vi "TCP Data Stream.vi"(0 "Address":string="localhost", 1 "Port":u16=2055 min=1025 step=1, 2 "Data IN":dbl[][](array[numeric]), 3 "String IN":string, 5 "Error IN":errorcluster, 6 "Mode":T1, 9 "Write String (F)":bool) -> (14 "Data OUT":dbl[][](array[numeric]), 15 "New Data?":bool, 16 "Connected?":bool, 17 "String OUT":string, 19 "Error OUT":errorcluster)   [LabVIEW 2019]
uses:
  Real-Time/Controls/TCP Data Stream Mode.ctl
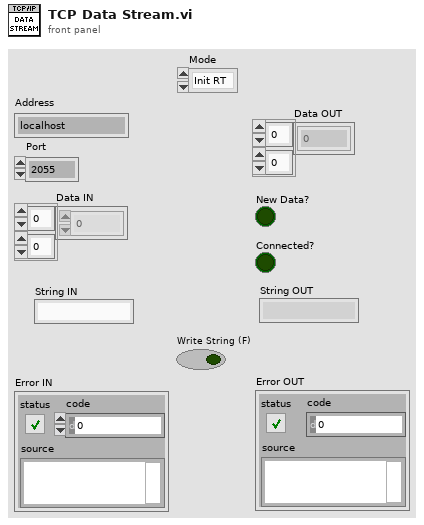
[diagram p1: front panel]
types:
  T1 = typedef "TCP Data Stream Mode.ctl" = enum16{"Init RT", "Init PC", "Connect RT", "Connect PC", "Write Data", "Read Data", "Close"}
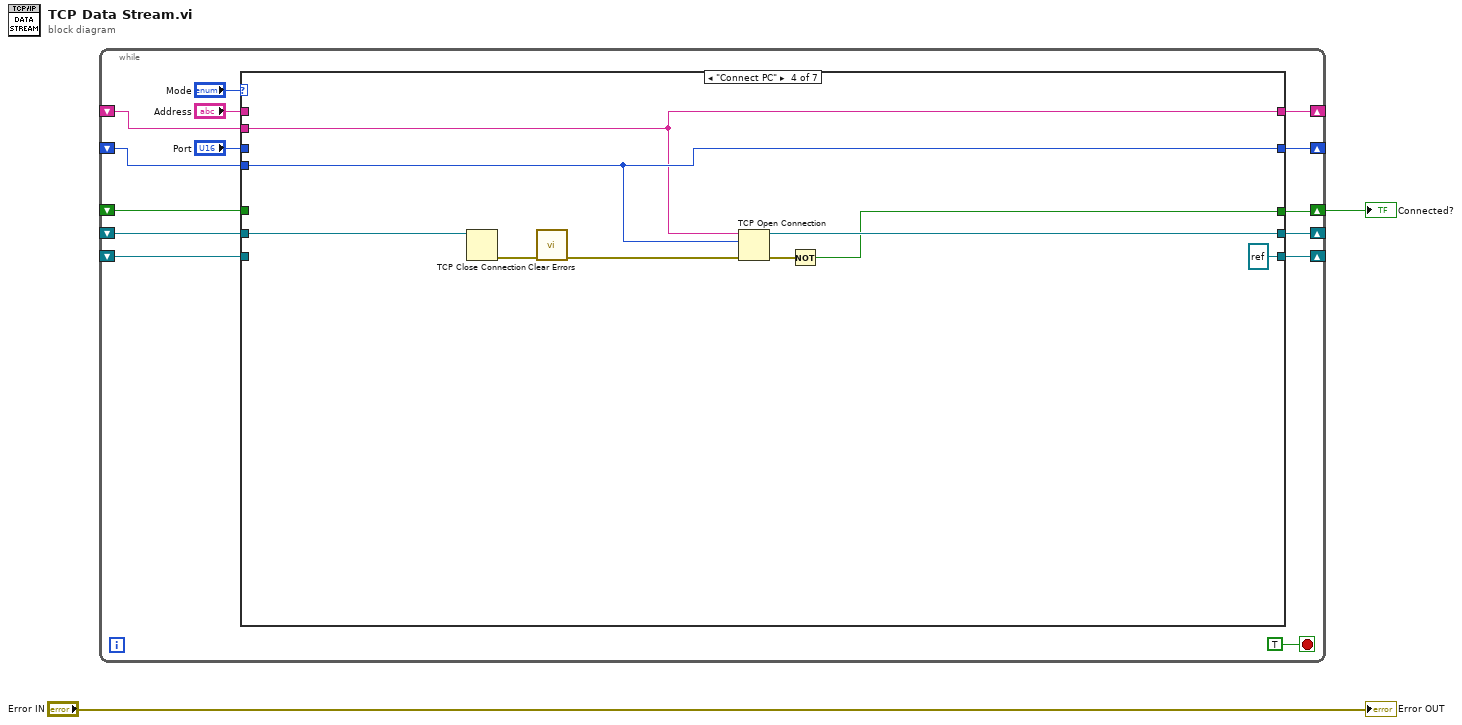
[diagram p0: block diagram]
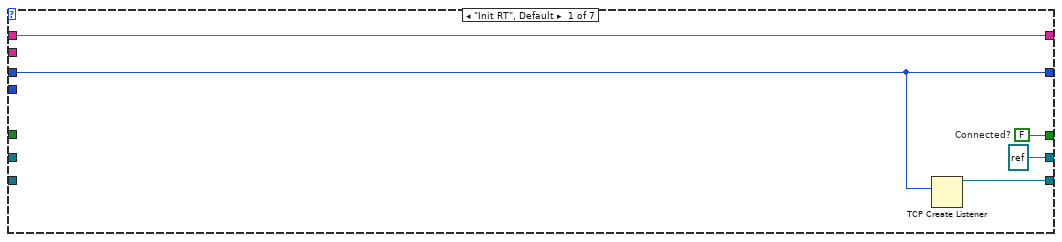
[diagram p2: hidden frame]
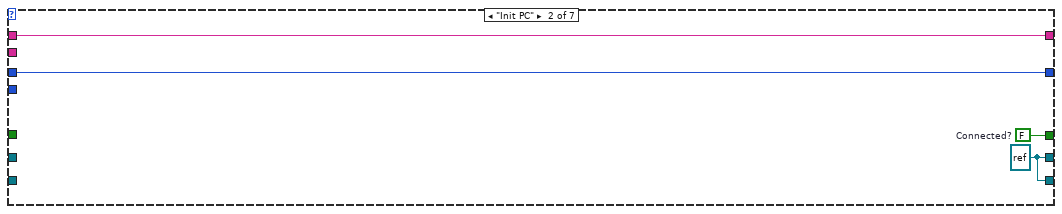
[diagram p3: hidden frame]
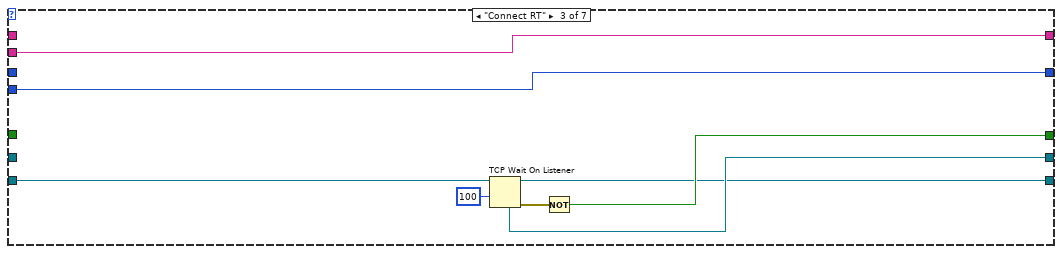
[diagram p4: hidden frame]
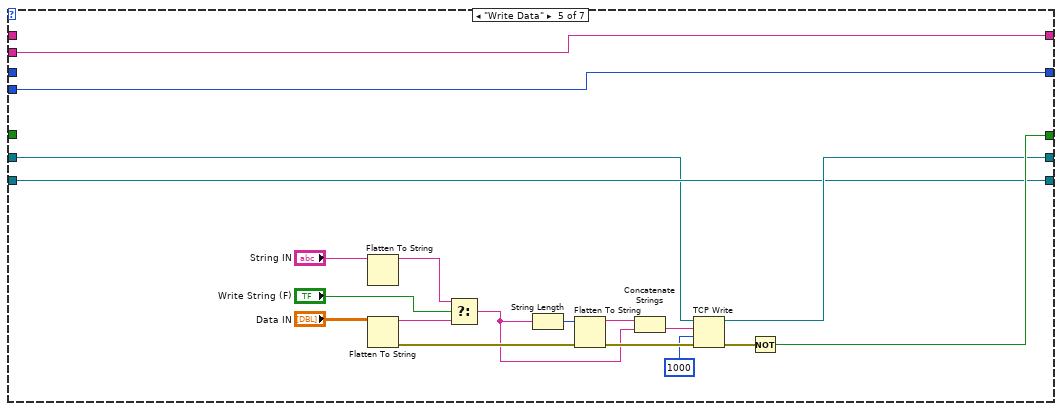
[diagram p5: hidden frame]
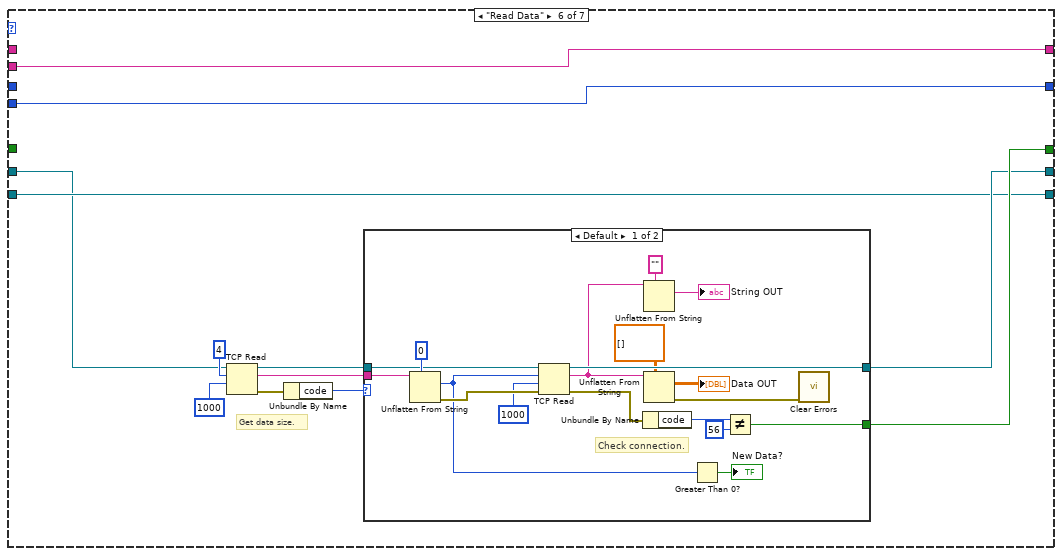
[diagram p6: hidden frame]
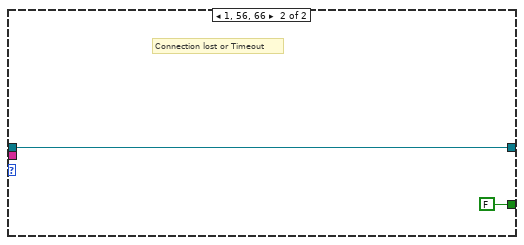
[diagram p7: hidden frame]
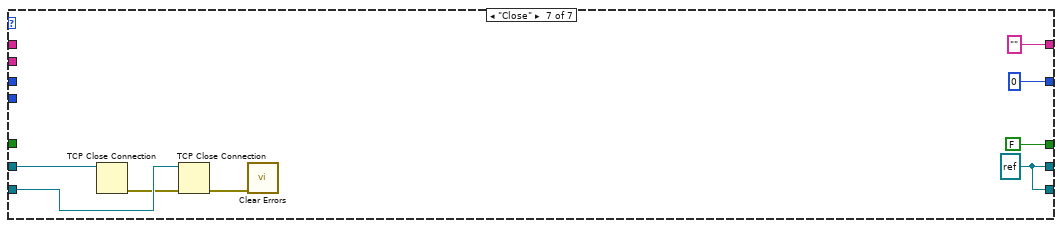
[diagram p8: hidden frame]
diagram:
  n1 = while {
    shift-right: [w13] -> _
    shift-left: _ -> [w8]
    shift-right: [w11] -> _
    shift-left: _ -> [w7]
    shift-right: [w10] -> w2
    shift-left: _ -> [w9]
    shift-right: [w6] -> _
    shift-left: _ -> [w5]
    shift-right: [w4] -> _
    shift-left: _ -> [w3]
    stop <- TRUE stop-if-true
    n2 = case shown="\"Connect PC\"" "Mode" {
      tunnel: [w21 w25 w27 w37 w60 w72 "" ("Address")] -> w13
      tunnel: "Address" -> [w21 w25 _ _ _ _ _]
      tunnel: [w19 w24 w28 w38 w61 w73 u16 0 ("Port")] -> w11
      tunnel: "Port" -> [w19 w24 _ _ _ _ _]
      tunnel: [w20 w23 w31 w40 w59 w71 FALSE ("Client")] -> w10
      tunnel: w9 -> [_ _ _ _ _ _ _]
      tunnel: w8 -> [_ _ w27 w37 w60 w72 _]
      tunnel: w7 -> [_ _ w28 w38 w61 w73 _]
      tunnel: [refnum<k5> refnum ("connection ID") w22 w30 w41 w58 w70 w98] -> w6
      tunnel: w5 -> [_ _ _ w36 w45 w62 w97]
      tunnel: [w17 w22 w29 refnum<k5> refnum ("connection ID") w57 w69 w98] -> w4
      tunnel: w3 -> [_ _ w32 _ w57 w69 w96]
      frame "Init RT", Default {
        w20 = FALSE  # Connected?
        n3 = TCP Create Listener(10:w19) -> (3:w17:refnum<k5>)  [unwired: 4 in, 2 out]
      }
      frame "Init PC" {
        w22 = refnum<k5> refnum ("connection ID")
        w23 = FALSE  # Connected?
      }
      frame "Connect RT" {
        n4 = TCP Wait On Listener(9:100 ("timeout ms (wait forever: -1)"), 11:w32) -> (0:w33:errorcluster, 3:w29:refnum<k5>, 4:w30:refnum<k5>)  [unwired: 2 in, 2 out]
        n5 = Not(x=w33) -> (.not. x?=w31:bool)
      }
      frame "Connect PC" {
        n6 = TCP Close Connection(connection ID=w36) -> (error out=w35:errorcluster)  [unwired: 2 in, 1 out]
        n7 = call <vilib>:"Clear Errors.vi"("error in (no error)"=w35) -> ("error out"=w34:errorcluster)  [unwired: 5 in, 1 out]
        n8 = TCP Open Connection(address=w37, remote port or service name=w38, error in (no error)=w34) -> (connection ID=w41:refnum<k5>, error out=w42:errorcluster)  [unwired: 2 in]
        n9 = Not(x=w42) -> (.not. x?=w40:bool)
      }
      frame "Write Data" {
        n10 = Flatten To String(anything="String IN") -> (data string=w47:string)  [unwired: 1 in, 4 out]
        n11 = Flatten To String(anything="Data IN") -> (data string=w48:string, error out=w55:errorcluster)  [unwired: 1 in, 3 out]
        n12 = Select(t=w47, s="Write String (F)", f=w48) -> (s? t:f=w46:string)
        n13 = String Length(string=w46) -> (length=w53:i32)
        n14 = Flatten To String(anything=w53, error in (no error)=w55) -> (data string=w54:string, error out=w52:errorcluster)  [unwired: 3 out]
        n15 = Concatenate Strings(w54, w46) -> (w51:string)
        n16 = TCP Write(connection ID=w45, data in=w51, error in (no error)=w52, 9:1000 ("timeout ms (25000)")) -> (connection ID out=w58:refnum<k5>, error out=w56:errorcluster)  [unwired: 1 out]
        n17 = Not(x=w56) -> (.not. x?=w59:bool)
      }
      frame "Read Data" {
        # "Get data size."
        n18 = TCP Read(connection ID=w62, bytes to read=4, 9:1000 ("timeout ms (25000)")) -> (connection ID out=w67:refnum<k5>, data out=w66:string, error out=w65:errorcluster)  [unwired: 1 in, 1 out]
        n19 = Unbundle By Name(w65) -> ("code"=w64:i32)
        n20 = case shown="Default" w64 {
          tunnel: [w78 FALSE] -> w71
          tunnel: [w84 w93] -> w70
          tunnel: w67 -> [w89 w93]
          tunnel: w66 -> [w88 _]
          frame Default {
            # "Check connection."
            n21 = Unflatten From String(type=0 ("bytes to read"), binary string=w88) -> (value=w81:i32, error out=w91:errorcluster)  [unwired: 2 in, 2 out]
            n22 = TCP Read(connection ID=w89, bytes to read=w81, error in (no error)=w91, 9:1000 ("timeout ms (25000)")) -> (connection ID out=w84:refnum<k5>, data out=w76:string, error out=w85:errorcluster)  [unwired: 1 out]
            n23 = Unbundle By Name(w85) -> ("code"=w87:i32)
            n24 = Unflatten From String(type="", binary string=w76) -> (value=→"String OUT":string)  [unwired: 1 in, 4 out]
            n25 = Unflatten From String(type=dbl[][] [] ("Data OUT"), binary string=w76) -> (value=→"Data OUT":dbl[][], error out=w79:errorcluster)  [unwired: 1 in, 3 out]
            n26 = Greater Than 0?(x=w81) -> (x > 0?=→"New Data?":bool)
            n27 = Not Equal?(x=w87, y=56) -> (x != y?=w78:bool)
            n28 = call <vilib>:"Clear Errors.vi"("error in (no error)"=w79) -> ()  [unwired: 5 in, 2 out]
          }
          frame 1, 56, 66 {
            # "Connection lost or Timeout"
          }
        }
      }
      frame "Close" {
        w98 = refnum<k5> refnum ("connection ID")
        n29 = TCP Close Connection(connection ID=w97) -> (error out=w95:errorcluster)  [unwired: 2 in, 1 out]
        n30 = TCP Close Connection(connection ID=w96, error in (no error)=w95) -> (error out=w94:errorcluster)  [unwired: 1 in, 1 out]
        n31 = call <vilib>:"Clear Errors.vi"("error in (no error)"=w94) -> ()  [unwired: 5 in, 2 out]
      }
    }
  }
  "Connected?" <- w2
  "Error OUT" <- "Error IN"
